vi "GV Config.vi"() -> ()   [LabVIEW 2018]
panel:
  in  "Sample period":dbl=0.1
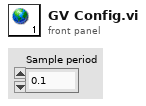
[diagram p1: front panel]
diagram:
